vi "SetTarget.vi"(10 "AutoReadChannels":T1, 11 "ServerData":T3) -> ()   [LabVIEW 2010]
uses:
  Ctrls/ServerData.ctl
  Ctrls/DeviceInfomation.ctl
  Ctrls/DeviceModel.ctl
  Ctrls/ChannelData.ctl
  Ctrls/ChannelType.ctl
  Ctrls/ChannelAccessType.ctl
  DeviceListChannelData.ctl
  AutoChannelData.ctl
  SubVIs/ModBUS Driver/Private/MBDRV_Action.ctl
  SubVIs/ModBUS Driver/Private/MBDRV_Command Data.ctl
  MonitorServer.lvlib
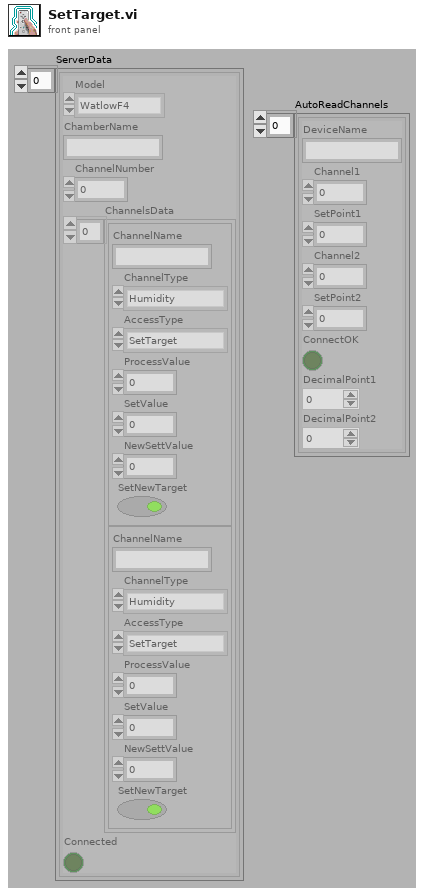
[diagram p1: front panel]
types:
  T1 = typedef "MonitorServer.lvlib/DeviceListChannelData.ctl" = T2[]
  T2 = typedef "MonitorServer.lvlib/AutoChannelData.ctl" = cluster{"DeviceName":string, "Channel1":dbl, "SetPoint1":dbl, "Channel2":dbl, "SetPoint2":dbl, "ConnectOK":bool, "DecimalPoint1":i16, "DecimalPoint2":i16}
  T3 = typedef "ServerData.ctl" = T4[]
  T4 = typedef "DeviceInfomation.ctl" = cluster{"Model":T5, "ChamberName":string, "ChannelNumber":i32, "ChannelsData":T6[], "Connected":bool}
  T5 = typedef "DeviceModel.ctl" = enum16{"WatlowF4", "CenterOne", "DCP551", "DPR250"}
  T6 = typedef "ChannelData.ctl" = cluster{"ChannelName":string, "ChannelType":T7, "AccessType":T8, "ProcessValue":dbl, "SetValue":dbl, "NewSettValue":dbl, "SetNewTarget":bool}
  T7 = typedef "ChannelType.ctl" = enum16{"Temperature", "Humidity"}
  T8 = typedef "ChannelAccessType.ctl" = enum16{"ReadOnly", "SetTarget"}
  T9 = typedef "MBDRV_Action.ctl" = enum16{"Write", "Read"}
  T10 = typedef "MBDRV_Command Data.ctl" = cluster{"Action":T9, "Com Port":string, "Register Address":u16, "Data To Write/Num To Read":i16}
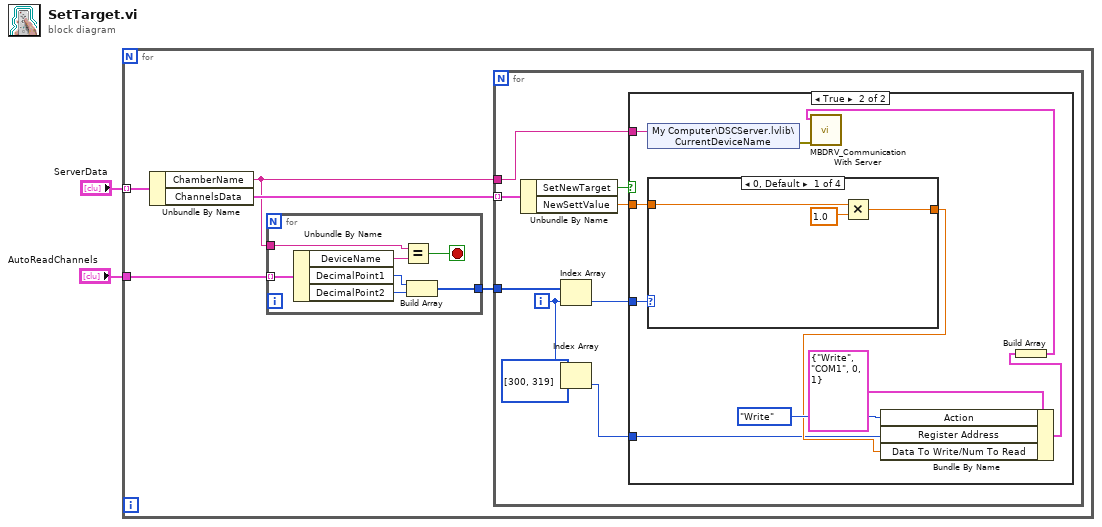
[diagram p0: block diagram]
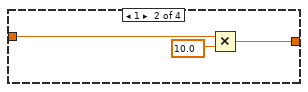
[diagram p3: hidden frame]
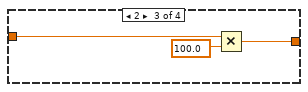
[diagram p4: hidden frame]
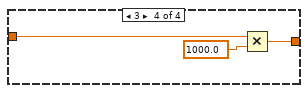
[diagram p5: hidden frame]
diagram:
  n1 = for {
    tunnel: "ServerData" -> [w7] mode=indexing
    tunnel: "AutoReadChannels" -> [w5]
    n2 = Unbundle By Name(w7) -> ("ChamberName"=w3:string, "ChannelsData"=w6:T6[])
    n3 = for {
      tunnel: w5 -> [w14] mode=indexing
      tunnel: [w11] -> w4
      tunnel: w3 -> [w9]
      stop <- w8 stop-if-true
      n4 = Unbundle By Name(w14) -> ("DeviceName"=w10:string, "DecimalPoint1"=w13:i16, "DecimalPoint2"=w12:i16)
      n5 = Equal?(x=w9, y=w10) -> (x = y?=w8:bool)
      n6 = Build Array(w13, w12) -> (w11:i16[])
    }
    n7 = for {
      tunnel: w6 -> [w23] mode=indexing
      tunnel: w3 -> [w20]
      tunnel: w4 -> [w19]
      i -> [w17]
      n8 = Unbundle By Name(w23) -> ("SetNewTarget"=w22:bool, "NewSettValue"=w21:dbl)
      n9 = Index Array(array=w19, index=w17) -> (element=w18:i16)
      n10 = Index Array(array=i16[] [300, 319], index=w17) -> (element=w15:i16)
      n11 = case shown="True" w22 {
        tunnel: w21 -> [_ w31]
        tunnel: w20 -> [_ w33]
        tunnel: w18 -> [_ w32]
        tunnel: w15 -> [_ w24]
        frame False {
        }
        frame True {
          n12 = shared-variable "My Computer\\DSCServer.lvlib\\CurrentDeviceName"(w33) -> (error out=w30:errorcluster)  [unwired: 1 in]
          n13 = case shown="0, Default" w32 {
            tunnel: [w35 w38 w41 w44] -> w25
            tunnel: w31 -> [w34 w37 w40 w43]
            frame 0, Default {
              n14 = Multiply(x=w34, y=1.0) -> (x*y=w35:dbl)
            }
            frame 1 {
              n15 = Multiply(x=w37, y=10.0) -> (x*y=w38:dbl)
            }
            frame 2 {
              n16 = Multiply(x=w40, y=100.0) -> (x*y=w41:dbl)
            }
            frame 3 {
              n17 = Multiply(x=w43, y=1000.0) -> (x*y=w44:dbl)
            }
          }
          n18 = Bundle By Name(cluster=T10 {"Action"=enum."Write", "Com Port"="COM1", "Register Address"=0, "Data To Write/Num To Read"=1} ("Command"), "Action"=MBDRV_Action."Write", "Register Address"=w24, "Data To Write/Num To Read"=w25) -> (w27:T10)
          n19 = Build Array(w27) -> (w26:T10[])
          n20 = call "MBDRV_Communication With Server.vi"("error in (no error)"=w30, "Write To PLC"=w26) -> ()  [unwired: 8 in, 2 out]
        }
      }
    }
  }
